vi "DCA Convert 1.10 - 1.11 to 2.0 - 2.1.vi"(0 "DCA 1.10 - 1.11 Test Parameters":T12={"Stimulus"={"Use Instrument"=FALSE, "Normalize"=FALSE, "Blank Screen"=FALSE, "Measurement Type"=enum."Voltage DC", "Range"=enum."Auto", "Resolution"=enum."Auto"}, "Measurement"={"Topology"=enum."PI-Network", "Lock Topology"=FALSE, "ATTN Calc"=enum."Power", "Zo"=50.0}, "Limits"=[]}) -> (2 "DCA 2.0 - 2.1 Test Parameters":T1={"Stimulus"={"Use Instrument"=FALSE, "Normalize"=FALSE, "Blank Screen"=FALSE, "Measurement Type"=enum."Diode", "Range"=enum."Auto", "Resolution"=enum."Auto"}, "Measurement"={"Topology"=enum."PI-Network", "Lock Topology"=FALSE, "ATTN Calc"=enum."Power", "Zo"=50.0}, "Limits"=[], "Normalization"={"Normalized?"=FALSE, "Rab Value"=0.0, "Rac Value"=0.0, "Rbc Value"=0.0}})   [LabVIEW 2011]
uses:
  TypeDefs/DCA Test Parameters v1.10-1.11.ctl
  TypeDefs/DCA Stimulus Parameters.ctl
  TypeDefs/DCA Measurement Cluster.ctl
  TypeDefs/DCA Topology.ctl
  TypeDefs/DCA Attenuation Calculation.ctl
  TypeDefs/DCA Limit.ctl
  TypeDefs/DCA Limit Quantity.ctl
  TypeDefs/DCA Limit Comparison.ctl
  TypeDefs/DCA Limit Operation.ctl
  Test Referential Limit.ctl
  TypeDefs/DCA Test Parameters.ctl
  TypeDefs/DCA Calibration State.ctl
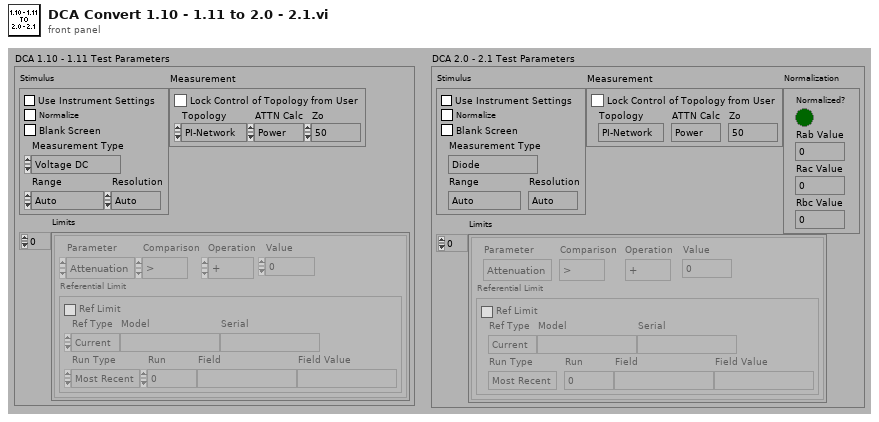
[diagram p1: front panel]
types:
  T1 = typedef "DCA Test Parameters.ctl" = cluster{"Stimulus":T2, "Measurement":T3, "Limits":T6[], "Normalization":T11}
  T2 = typedef "DCA Stimulus Parameters.ctl" = cluster{"Use Instrument":bool, "Normalize":bool, "Blank Screen":bool, "Measurement Type":enum16{"Voltage DC", "Voltage DC Ratio", "Voltage AC", "Current DC", "Current AC", "Resistance", "Fresistance", "Frequency", "Period", "Continuity", "Diode"}, "Range":enum16{"Auto", "Minimum", "Maximum", "100", "1,000", "10,000", "100,000", "1,000,000", "10,000,000", "100,000,000"}, "Resolution":enum16{"Auto", "4 1/2", "5 1/2", "6 1/2"}}
  T3 = typedef "DCA Measurement Cluster.ctl" = cluster{"Topology":T4, "Lock Topology":bool, "ATTN Calc":T5, "Zo":dbl}
  T4 = typedef "DCA Topology.ctl" = enum32{"PI-Network", "T-Network"}
  T5 = typedef "DCA Attenuation Calculation.ctl" = enum32{"Power", "Voltage"}
  T6 = typedef "DCA Limit.ctl" = cluster{"Parameter":T7, "Comparison":T8, "Operation":T9, "Value":dbl, "Referential Limit":T10}
  T7 = typedef "DCA Limit Quantity.ctl" = enum16{"Attenuation", "Zin", "Zout", "R1", "R2", "R3", "Rab", "Rac", "Rbc"}
  T8 = typedef "DCA Limit Comparison.ctl" = enum16{">", ">=", "<", "<="}
  T9 = typedef "DCA Limit Operation.ctl" = enum16{"+", "-"}
  T10 = typedef "Test Referential Limit.ctl" = cluster{"Ref Limit":bool, "Ref Type":enum16{"Current", "Specify"}, "Model":string, "Serial":string, "Run Type":enum16{"Most Recent", "Run #", "Match Field"}, "Run":i32, "Field":string, "Field Value":string}
  T11 = typedef "DCA Calibration State.ctl" = cluster{"Normalized?":bool, "Rab Value":dbl, "Rac Value":dbl, "Rbc Value":dbl}
  T12 = typedef "DCA Test Parameters v1.10-1.11.ctl" = cluster{"Stimulus":T2, "Measurement":T3, "Limits":T6[]}
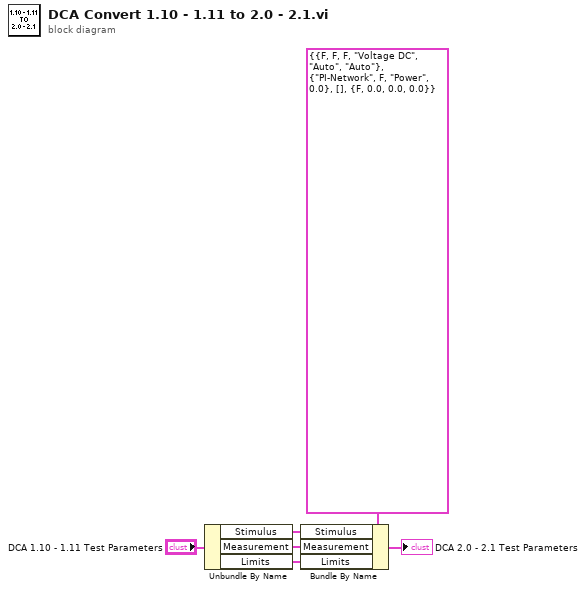
[diagram p0: block diagram]
diagram:
  n1 = Unbundle By Name("DCA 1.10 - 1.11 Test Parameters") -> ("Stimulus"=w4:T2, "Measurement"=w1:T3, "Limits"=w3:T6[])
  n2 = Bundle By Name(cluster=T1 {"Stimulus"={"Use Instrument"=FALSE, "Normalize"=FALSE, "Blank Screen"=FALSE, "Measurement Type"=enum."Voltage DC", "Range"=enum."Auto", "Resolution"=enum."Auto"}, "Measurement"={"Topology"=enum."PI-Network", "Lock Topology"=FALSE, "ATTN Calc"=enum."Power", "Zo"=0.0}, "Limits"=[], "Normalization"={"Normalized?"=FALSE, "Rab Value"=0.0, "Rac Value"=0.0, "Rbc Value"=0.0}} ("DCA 1.9 Test Parameters"), "Stimulus"=w4, "Measurement"=w1, "Limits"=w3) -> (→"DCA 2.0 - 2.1 Test Parameters":T1)
